vi "Save Recall State.vi"(8 "error in":errorcluster, 9 "State Number":i32, 10 "State":i32(ring) items=["Save", "Recall"], 11 "Instrument Handle In":i32) -> (0 "error out":errorcluster, 3 "Instrument Handle Out":i32)   [LabVIEW 8.6, in "ZTScopeM.lvlib"]
doc: "Save or recall an instrument state from non-volatile memory."
uses:
  ZTScopeM.lvlib
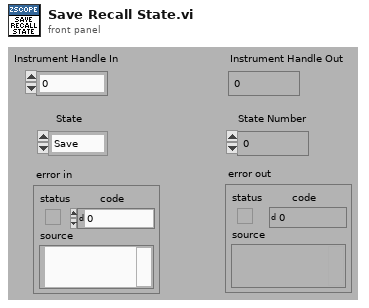
[diagram p1: front panel]
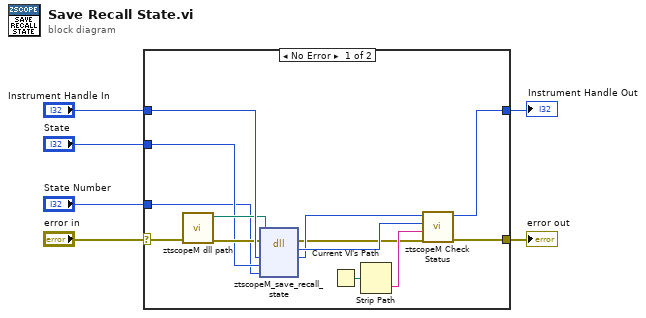
[diagram p0: block diagram]
diagram:
  n1 = case shown="No Error" "error in" {
    selector: "error in" -> [w12 w21]
    tunnel: [w14 w21] -> w3
    tunnel: "Instrument Handle In" -> [w19 w20]
    tunnel: [w13 w20] -> w5
    tunnel: "State" -> [w8 _]
    tunnel: "State Number" -> [w7 _]
    frame #0 {
      n2 = call "ztscopeM dll path.vi"("error in (no error)"=w12) -> ("error out"=w10:errorcluster, "<instrument>.dll path"=w11:path)  [unwired: 9 in]
      n3 = dll-call lib="C:/Program Files (x86)/National Instruments/LabVIEW 2013/instr.lib/ztscopem/ztscopeM.dll" fn="ztscopeM_save_recall_state"(path in=w11, error in=w10, "instrumentHandle"=w19, "state"=w8, "state_number"=w7) -> (error out=w9:errorcluster, w16:i32, "instrumentHandle"=w15:i32)  [unwired: 3 in, 1 out]
      n4 = Current VI's Path() -> (path=w18:path)
      n5 = Strip Path(path=w18) -> (name=w17:string)  [unwired: 1 out]
      n6 = call "ztscopeM Check Status.vi"("error in"=w9, "name of VI"=w17, "status (return code)"=w16, "instrument handle in"=w15) -> ("error out"=w14:errorcluster, "instrument handle out"=w13:i32)  [unwired: 2 in]
    }
    frame #1 {
    }
  }
  "Instrument Handle Out" <- w5
  "error out" <- w3
